vi "D2SParser - Private - Helper - Read ASCII.vi"(8 "error in (no error)":errorcluster, 9 "# Characters":i32, 10 "Position":i64, 11 "D2SParser in":refnum<class "D2SParser.lvclass">) -> (0 "error out":errorcluster, 2 "ASCII":string, 3 "D2SParser out":refnum<class "D2SParser.lvclass">)   [LabVIEW 2015, in "D2SParser.lvclass"]
uses:
  D2SParser.lvclass
  D2SParser.lvclass/D2SParser.ctl
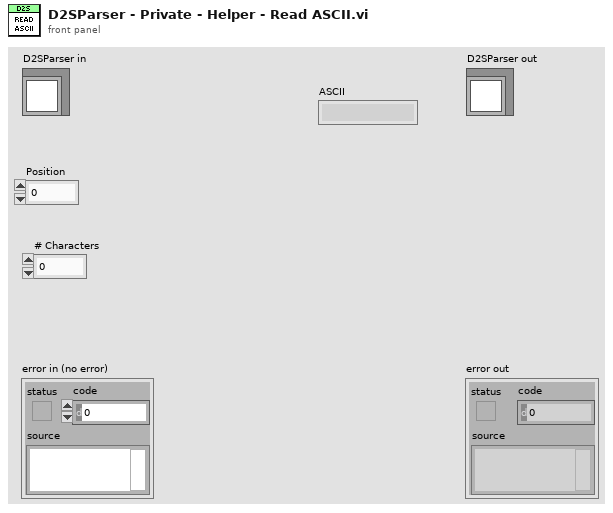
[diagram p1: front panel]
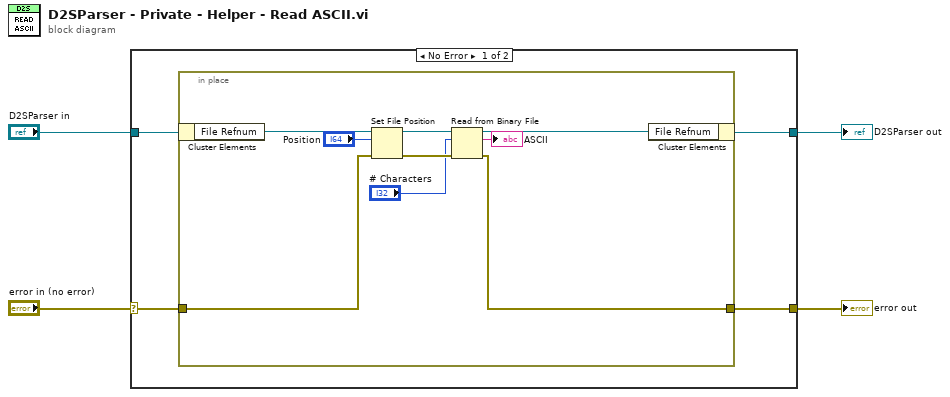
[diagram p0: block diagram]
diagram:
  n1 = case shown="No Error" "error in (no error)" {
    selector: "error in (no error)" -> [w7 w19]
    tunnel: [w6 w19] -> w3
    tunnel: [w5 w18] -> w1
    tunnel: "D2SParser in" -> [w8 w18]
    frame No Error {
      n2 = in-place {
        in-place-border: w7 -> [w13]
        in-place-border: [w11] -> w6
        n3 = in-place-cluster #1(w8) -> ("File Refnum"=w15:refnum<file>)
        n4 = Set File Position(offset (in bytes) (0)="Position", refnum=w15, error in=w13) -> (refnum out=w16:refnum<file>, error out=w17:errorcluster)  [unwired: 1 in]
        n5 = Read from Binary File(8:w17, 10:"# Characters", 11:w16) -> (0:w11:errorcluster, 2:→"ASCII":string, 3:w14:refnum<file>)  [unwired: 3 in, 1 out]
        n6 = in-place-cluster #1("File Refnum"=w14) -> (w5:refnum<class "D2SParser.lvclass">)
      }
    }
    frame Error {
    }
  }
  "error out" <- w3
  "D2SParser out" <- w1
